vi "Leap-suona.vi"() -> ()   [LabVIEW 2014]
uses:
  <vilib>/sound2/lvsound2.llb/Sampling Mode.ctl
  <vilib>/sound2/lvsound2.llb/Sound Data Format.ctl
  <vilib>/sound2/lvsound2.llb/Sound Output Set Volume (Single).vi
  <vilib>/sound2/lvsound2.llb/Sound Output Write (DBL Single).vi
panel:
  out "Key tap":string[](array[string])
  in  "Device ID":u32
  in  "Stop":bool
  out "Generated Sound":waveform(dbl)(graph)
  in  "Volume":dbl(slide)=50.0 scale=0.0..100.0
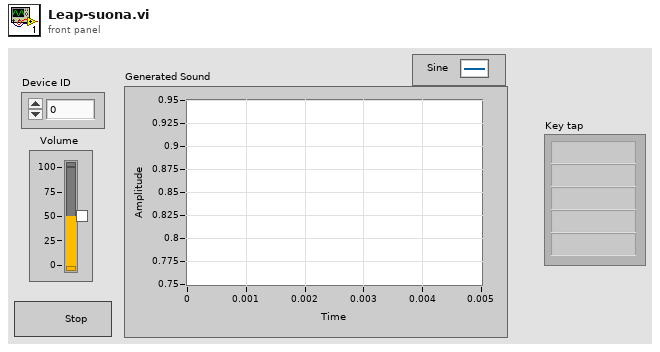
[diagram p1: front panel]
types:
  T1 = typedef "Sound Data Format.ctl" = cluster{"sample rate (S/s)":dbl, "number of channels":i32, "bits per sample":i32}
  T2 = typedef "Sampling Mode.ctl" = i32
  T3 = typedef "Sound Output Task ID.ctl" = u32
  T4 = typedef "Leap Handle.ctl" = cluster{"LeapCSharp":refnum<k24>}
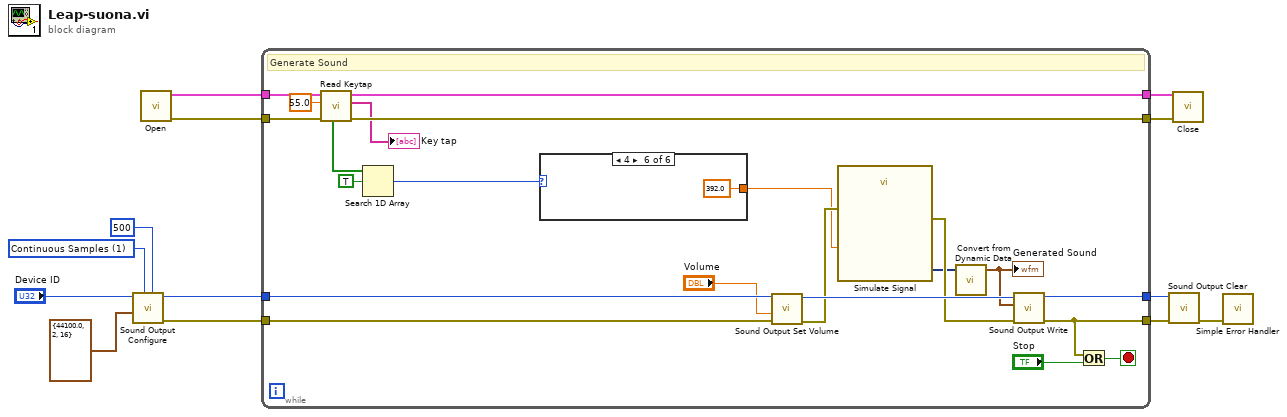
[diagram p0: block diagram]
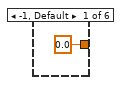
[diagram p2: hidden frame]
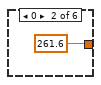
[diagram p3: hidden frame]
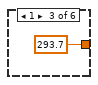
[diagram p4: hidden frame]
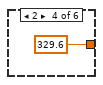
[diagram p5: hidden frame]
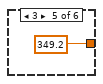
[diagram p6: hidden frame]
diagram:
  w8 = T2 1 items=["Finite Samples", "Continuous Samples"] ("sample mode")
  n1 = call <vilib>:"Sound Output Configure.vi"("number of samples/ch"=500 ("Number of Samples/ch"), "sample mode"=w8, "sound format"=T1 {"sample rate (S/s)"=44100.0, "number of channels"=2, "bits per sample"=16} ("Sound Format"), "device ID"="Device ID") -> ("error out"=w13:errorcluster, "task ID"=w12:T3)  [unwired: 6 in]
  n2 = call "Open.vi"() -> ("Error Out"=w3:errorcluster, "Leap Handle"=w4:T4)  [unwired: 10 in]
  n3 = while {
    tunnel: w12 -> [w30]
    tunnel: [w35] -> w10
    tunnel: w13 -> [w32]
    tunnel: [w28] -> w11
    tunnel: w4 -> [w22]
    tunnel: w3 -> [w21]
    tunnel: [w20] -> w2
    tunnel: [w19] -> w1
    stop <- w33 stop-if-true
    # "Generate Sound"
    n4 = call "Read Keytap.vi"("Error In"=w21, "Key Tap Thresh"=sgl 55.0, "Leap Handle In"=w22) -> ("Error Out"=w19:errorcluster, "Key tap"=→"Key tap":string[], "Leap Handle Out"=w20:T4, "Index Array"=w15:bool[])  [unwired: 2 in, 2 out]
    n5 = Search 1D Array(1D array=w15, element=TRUE) -> (index of element=w16:i32)  [unwired: 1 in]
    n6 = case shown="4" w16 {
      tunnel: [0.0 ("Volume") 261.6 ("Volume") 293.7 ("Volume") 329.6 ("Volume") 349.2 ("Volume") 392.0 ("Volume")] -> w23
      frame -1, Default {
      }
      frame 0 {
      }
      frame 1 {
      }
      frame 2 {
      }
      frame 3 {
      }
      frame 4 {
      }
    }
    n7 = call-poly <vilib>:"Sound Output Set Volume.vi"("error in (no error)"=w32, "volume"="Volume", "task ID"=w30) -> ("error out"=w26:errorcluster, "task ID out"=w31:T3)  [unwired: 7 in]
    n8 = call "Simulate Signal"("Frequency"=w23, "error in (no error)"=w26) -> ("Sine"=w24:dynamicdata, "error out"=w25:errorcluster)  [unwired: 12 in]
    n9 = call "Convert from Dynamic Data"("Dynamic Data Type"=w24) -> ("Waveform"=w27:waveform(dbl))  [unwired: 3 in]
    "Generated Sound" <- w27
    n10 = call-poly <vilib>:"Sound Output Write.vi"("error in (no error)"=w25, "data"=w27, "task ID"=w31) -> ("error out"=w28:errorcluster, "task ID out"=w35:T3)  [unwired: 7 in]
    n11 = Or(x=w28, y="Stop") -> (x .or. y?=w33:bool)
  }
  n12 = call <vilib>:"Sound Output Clear.vi"("error in (no error)"=w11, "task ID"=w10) -> ("error out"=w6:errorcluster)  [unwired: 9 in]
  n13 = call "Close.vi"("Error In"=w1, "Leap Handle"=w2) -> ()  [unwired: 9 in, 1 out]
  n14 = call <vilib>:"Simple Error Handler.vi"("error in (no error)"=w6) -> ()  [unwired: 4 in, 5 out]
